vi "PH_OceanOpticsSpectrometer.PC Set Trigger.vi"(0 "VI in":refnum<vi>, 2 "Wanted Trigger":T1, 5 "error in (no error)":errorcluster) -> (14 "VI out":refnum<vi>, 19 "error out":errorcluster)   [LabVIEW 2014, in "PH_OceanOpticsSpectrometer.lvlib"]
doc: "This VI sets the wanted trigger setting to hardware and stores it at own attributes."
uses:
  PH_OceanOpticsSpectrometer.lvlib
  PH_OceanOpticsSpectrometer.Trigger.ctl
  non_GPL/instr.lib/Ocean Optics 2000 4000/Ocean Optics 2000 4000 - Driver np.lvlib
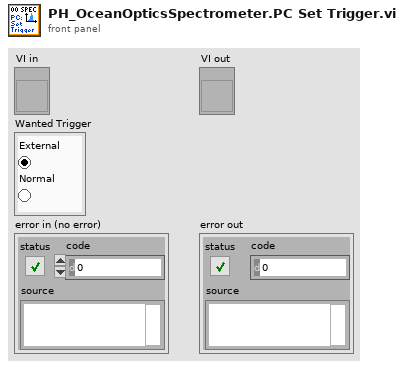
[diagram p1: front panel]
types:
  T1 = typedef "PH_OceanOpticsSpectrometer.lvlib/PH_OceanOpticsSpectrometer.Trigger.ctl" = enum32{"External", "Normal"}
  T2 = typedef "PH_OceanOpticsSpectrometer.lvlib/PH_OceanOpticsSpectrometer.i attribute.ctl" = cluster{"GUI Refs":cluster{"Delete":refnum<vi>, "Spectrum":refnum<vi>, "Display Width":refnum<vi>, "Display Center":refnum<vi>, "Save":refnum<vi>, "Integration time":refnum<vi>, "center wavelength":refnum<vi>, "width":refnum<vi>, "Wanted Trigger Mode":refnum<vi>, "Current Trigger Mode":refnum<vi>, "Trigger Info":refnum<vi>, "Model":refnum<vi>, "Driver":refnum<vi>, "Firmware":refnum<vi>}, "Display":cluster{"Width":dbl, "Center":dbl}, "VISA resource name":refnum<visa-resource-name>, "Integration time [ms]":cluster{"Current Value":u16, "Wanted Value":u16}, "Trigger":cluster{"Current value":T1, "Wanted value":T1}, "Default VISA Timeout":u32, "Last Data":cluster{"Wavelength Bins":dbl[], "Spectrum by Pixels":dbl[]}}
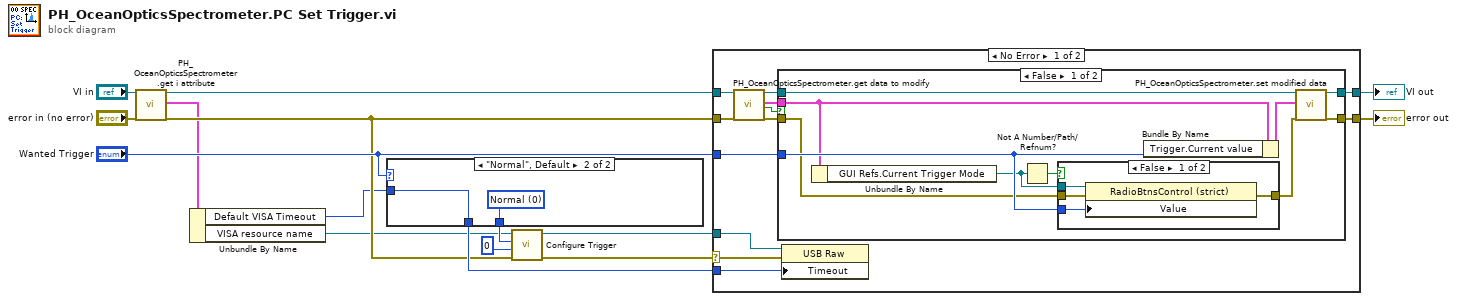
[diagram p0: block diagram]
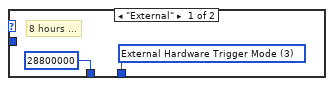
[diagram p2: hidden frame]
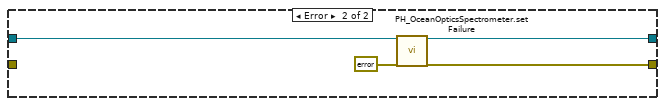
[diagram p5: hidden frame]
diagram:
  n1 = call "PH_OceanOpticsSpectrometer.get i attribute.vi"("i ref in"="VI in", "error in (no error)"="error in (no error)") -> ("i ref out"=w4:refnum<vi>, "i attribute"=w3:T2, "error out"=w6:errorcluster)  [unwired: 15 in]
  n2 = Unbundle By Name(w3) -> ("Default VISA Timeout"=w2:u32, "VISA resource name"=w1:refnum<visa-resource-name>)
  n3 = case shown="\"Normal\", Default" "Wanted Trigger" {
    tunnel: [w17 w19] -> w12
    tunnel: [u32 28800000 ("Default VISA Timeout") w18] -> w15
    tunnel: w2 -> [_ w18]
    frame "External" {
      w17 = u8 3 items=["Normal", "Software Trigger Mode", "External Sync Trigger Mode", "External Hardware Trigger Mode"] ("Trigger Type (0:Normal) 2")
      # "8 hours ..."
    }
    frame "Normal", Default {
      w19 = u8 0 items=["Normal", "Software Trigger Mode", "External Sync Trigger Mode", "External Hardware Trigger Mode"] ("Trigger Type (0:Normal) 2")
    }
  }
  n4 = call "Configure Trigger.vi"("error in (no error)"=w6, "Hardware Trigger Delay (0 s)"=u16 0, "Trigger Type (0:Normal)"=w12, "VISA resource name"=w1) -> ("error out"=w11:errorcluster, "VISA resource name out"=w14:refnum<visa-resource-name>)  [unwired: 6 in]
  n5 = case shown="No Error" w11 {
    selector: w11 -> [w20 _]
    tunnel: [w31 w50] -> w8
    tunnel: w6 -> [w25 _]
    tunnel: w4 -> [w27 w52]
    tunnel: [w26 w51] -> w9
    tunnel: "Wanted Trigger" -> [w30 _]
    tunnel: w14 -> [w22 _]
    tunnel: w15 -> [w21 _]
    frame No Error {
      n6 = call "PH_OceanOpticsSpectrometer.get data to modify.vi"("i ref in"=w27, "error in (no error)"=w25) -> ("i ref out"=w29:refnum<vi>, "i attribute"=w23:T2, "timed out"=w24:bool, "error out"=w28:errorcluster)  [unwired: 14 in]
      n7 = case shown="False" w24 {
        tunnel: [w35 w47] -> w31
        tunnel: w30 -> [w37 _]
        tunnel: w29 -> [w40 w48]
        tunnel: w28 -> [w34 w47]
        tunnel: [w38 w48] -> w26
        tunnel: w23 -> [w33 _]
        frame False {
          n8 = Unbundle By Name(w33) -> ("GUI Refs.Current Trigger Mode"=w32:refnum<vi>)
          n9 = Not A Number/Path/Refnum?(number/path/refnum=w32) -> (NaN/Path/Refnum?=w41:bool)
          n10 = case shown="False" w41 {
            tunnel: w32 -> [w44 _]
            tunnel: w34 -> [w45 w46]
            tunnel: [w43 w46] -> w36
            tunnel: w37 -> [w42 _]
            frame False {
              n11 = property class="RadioBtnsControl (strict)"(reference=w44, error in=w45, "Value"=w42) -> (error out=w43:errorcluster)  [unwired: 1 out]
            }
            frame True {
            }
          }
          n12 = Bundle By Name(cluster=w33, "Trigger.Current value"=w37) -> (w39:T2)
          n13 = call "PH_OceanOpticsSpectrometer.set modified data.vi"("i ref in"=w40, "i attribute"=w39, "error in (no error)"=w36) -> ("i ref out"=w38:refnum<vi>, "error out"=w35:errorcluster)  [unwired: 15 in]
        }
        frame True {
        }
      }
      n14 = property class="USB Raw"(reference=w22, error in=w20, "Timeout"=w21) -> ()  [unwired: 2 out]
    }
    frame Error {
      n15 = call "PH_OceanOpticsSpectrometer.set Failure.vi"("i ref in"=w52, "error IO"=errorcluster {"status"=FALSE, "code"=0, "source"=""}) -> ("i ref out"=w51:refnum<vi>, "error out"=w50:errorcluster)  [unwired: 16 in]
    }
  }
  "VI out" <- w9
  "error out" <- w8
